vi "Log Status Update.vi"(8 "error in (no error)":errorcluster, 10 "String":string, 11 "Controller in":refnum<class "Controller.lvclass">) -> (0 "error out":errorcluster, 3 "Controller out":refnum<class "Controller.lvclass">)   [LabVIEW 2017, in "Controller Actor.lvlib" / "Controller.lvclass"]
uses:
  Controller.lvclass
  User Interface/Messages/Update Status Display/Update Status Display.lvclass
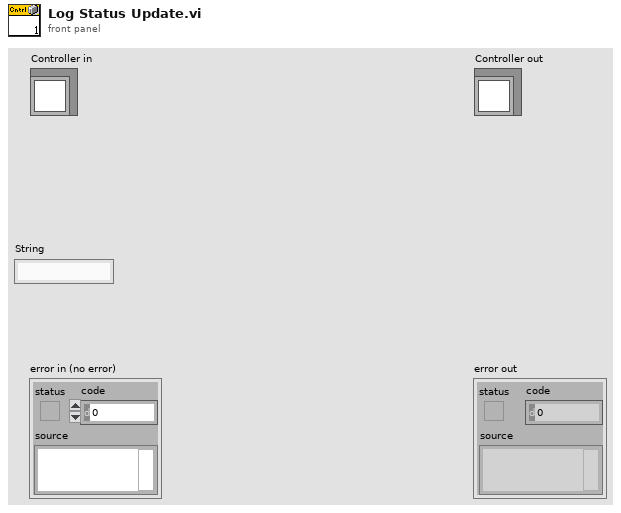
[diagram p1: front panel]
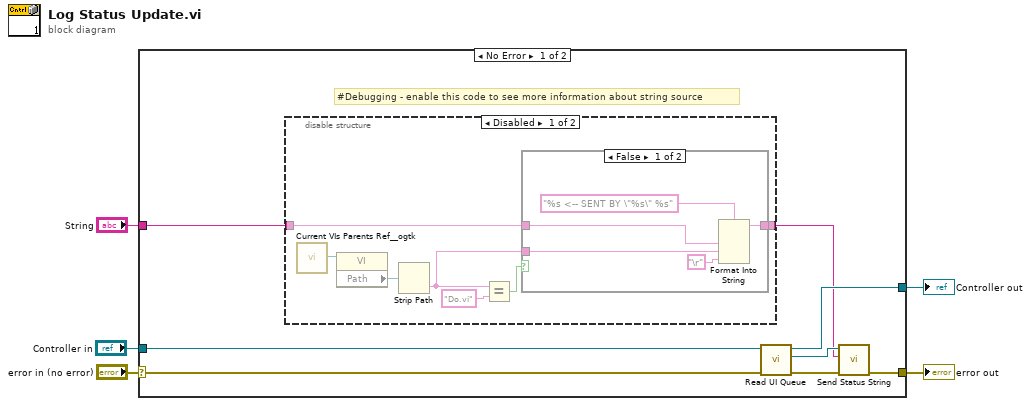
[diagram p0: block diagram]
diagram:
  n1 = case shown="No Error" "error in (no error)" {
    selector: "error in (no error)" -> [w10 w29]
    tunnel: [w11 w29] -> w4
    tunnel: [w12 w28] -> w2
    tunnel: "Controller in" -> [w13 w28]
    tunnel: "String" -> [w7 _]
    frame No Error {
      # "#Debugging - enable this code to see more information about string source"
      n2 = disable-structure shown="Disabled" {
        disable-tunnel: w7 -> [w15 w27]
        disable-tunnel: [w14 w27] -> w6
        frame Disabled {
          n3 = call <userlib>:"Current VIs Parents Ref__ogtk.vi"() -> ("Calling VI's Reference"=w17:refnum<vi>)  [unwired: 2 in]
          n4 = property class="VI"(reference=w17) -> ("Path"=w18:path)  [unwired: 1 in, 2 out]
          n5 = Strip Path(path=w18) -> (name=w19:string)  [unwired: 1 out]
          n6 = Equal?(x=w19, y="Do.vi") -> (x = y?=w16:bool)
          n7 = case shown="False" w16 {
            tunnel: w19 -> [w23 _]
            tunnel: w15 -> [w22 w26]
            tunnel: [w21 w26] -> w14
            frame False {
              n8 = Format Into String(format string="%s <-- SENT BY \"%s\" %s", w22, w23, "\r") -> (resulting string=w21:string)  [unwired: 2 in, 1 out]
            }
            frame True {
            }
          }
        }
        frame Enabled {
        }
      }
      n9 = call "Read UI Queue.vi"("error in (no error)"=w10, "UI Controller in"=w13) -> ("error out"=w8:errorcluster, "UI Queue"=w9:refnum<class "Message Enqueuer.lvclass">, "UI Controller out"=w12:refnum<class "Controller.lvclass">)  [unwired: 7 in]
      n10 = call "Send Status String.vi"("error in (no error)"=w8, "String"=w6, "Message Enqueuer in"=w9) -> ("error out"=w11:errorcluster)  [unwired: 7 in, 1 out]
    }
    frame Error {
    }
  }
  "error out" <- w4
  "Controller out" <- w2
